vi "GetRTMMenuReference.vi"(8 "error in":errorcluster, 11 "RTMFilePath":path) -> (0 "error out":errorcluster, 3 "RTMMenuReference":refnum<k9>)   [LabVIEW 2021, in "Menu.lvlib" / "Menu.lvclass"]
uses:
  Menu.lvclass
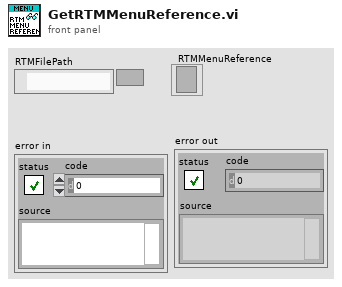
[diagram p1: front panel]
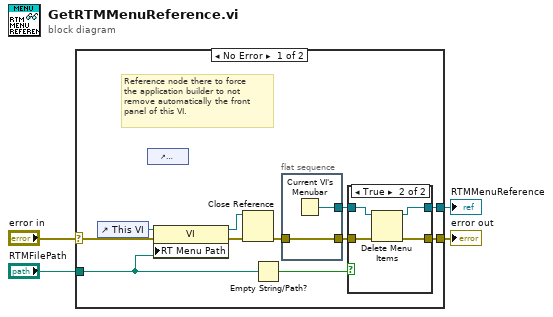
[diagram p0: block diagram]
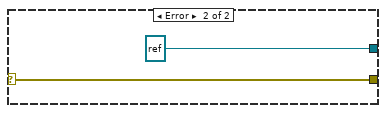
[diagram p3: hidden frame]
diagram:
  n1 = case shown="No Error" "error in" {
    selector: "error in" -> [w14 w24]
    tunnel: [w9 refnum<k9> refnum ("menu reference")] -> w4
    tunnel: [w8 w24] -> w3
    tunnel: "RTMFilePath" -> [w13 _]
    frame No Error {
      # "Reference node there to force\nthe application builder to not\nremove automatically the front\npanel of this VI."
      n2 = control-ref of="This VI"() -> (w7:refnum<vi>)
      n3 = control-ref of="RTMFilePath"() -> ()  [unwired: 1 out]
      n4 = property class="VI"(reference=w7, error in=w14, "RT Menu Path"=w13) -> (reference out=w5:refnum<vi>, error out=w6:errorcluster)
      n5 = Close Reference(reference=w5, error in (no error)=w6) -> (error out=w15:errorcluster)
      n6 = Empty String/Path?(string/path=w13) -> (empty?=w11:bool)
      n7 = flat-sequence {
        tunnel: [w23] -> w12
        tunnel: w15 -> [w23]
        tunnel: [w22] -> w10
        frame #0 {
          n8 = Current VI's Menubar() -> (w22:refnum<k9>)
        }
      }
      n9 = case shown="True" w11 {
        tunnel: w12 -> [w16 w20]
        tunnel: w10 -> [w17 w21]
        tunnel: [w17 w19] -> w9
        tunnel: [w16 w18] -> w8
        frame False {
        }
        frame True {
          n10 = Delete Menu Items(6:w20, 9:w21) -> (0:w18:errorcluster, 3:w19:refnum<k9>)  [unwired: 2 out]
        }
      }
    }
    frame Error {
    }
  }
  "RTMMenuReference" <- w4
  "error out" <- w3
